vi "有限步数转动.vi"(8 "error in (no error)":errorcluster caption="错误输入（无错误）", 10 "samples per channel":i32=1000 caption="脉冲数", 11 "Hardware Resources in":T1 caption="硬件资源输入") -> (0 "error out":errorcluster caption="错误输出", 3 "Hardware Resources out":T1 caption="硬件资源输出")   [LabVIEW 2015, in "Action.lvlib"]
doc: "初始化硬件引用。"
uses:
  Action.lvlib
  <vilib>/DAQmx/create/channels.llb/DAQmx Create Channel (CO-Pulse Generation-Frequency).vi
  <vilib>/DAQmx/configure/timing.llb/DAQmx Timing (Implicit).vi
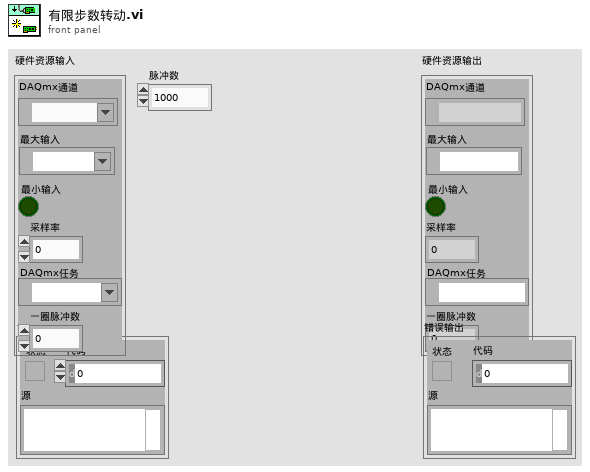
[diagram p1: front panel]
types:
  T1 = typedef "Action.lvlib/电机控制设置.ctl" = cluster{"counter":tag, "方向端口":tag, "当前方向":bool, "频率":dbl, "DAQmx Task":refnum<k21>, "一圈脉冲数":i32}
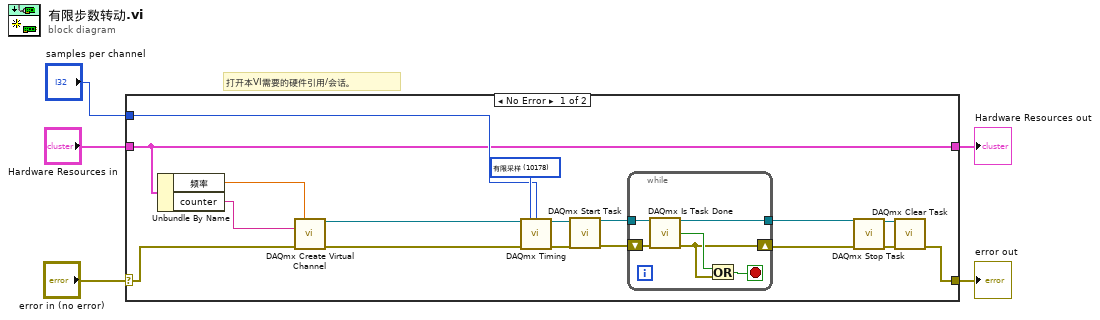
[diagram p0: block diagram]
diagram:
  # "打开本VI需要的硬件引用/会话。"
  n1 = case shown="No Error" "error in (no error)" {
    selector: "error in (no error)" -> [w6 w29]
    tunnel: [w20 w29] -> w4
    tunnel: "Hardware Resources in" -> [w15 w30]
    tunnel: [w15 w30] -> w2
    tunnel: "samples per channel" -> [w16 _]
    frame No Error {
      w17 = 10178 items=["有限采样"=10178, "连续采样"=10123, "硬件定时单点"=12522] ("sample mode")
      n2 = Unbundle By Name(w15) -> ("频率"=w18:dbl, "counter"=w19:tag)
      n3 = call-poly <vilib>:"DAQmx Create Virtual Channel.vi"("frequency"=w18, "counter"=w19, "error in"=w6) -> ("task out"=w8:refnum<k21>, "error out"=w7:errorcluster)  [unwired: 11 in]
      n4 = call-poly <vilib>:"DAQmx Timing.vi"("task/channels in"=w8, "sample mode"=w17, "samples per channel"=w16, "error in"=w7) -> ("task out"=w14:refnum<k21>, "error out"=w13:errorcluster)  [unwired: 10 in]
      n5 = call <vilib>:"DAQmx Start Task.vi"("task/channels in"=w14, "error in"=w13) -> ("task out"=w12:refnum<k21>, "error out"=w11:errorcluster)  [unwired: 12 in]
      n6 = while {
        tunnel: w12 -> [w28]
        shift-right: [w24] -> w9
        shift-left: w11 -> [w27]
        tunnel: [w23] -> w10
        stop <- w25 stop-if-true
        n7 = call <vilib>:"DAQmx Is Task Done.vi"("task/channels in"=w28, "error in"=w27) -> ("task out"=w23:refnum<k21>, "task done?"=w26:bool, "error out"=w24:errorcluster)  [unwired: 11 in]
        n8 = Or(x=w26, y=w24) -> (x .or. y?=w25:bool)
      }
      n9 = call <vilib>:"DAQmx Stop Task.vi"("task/channels in"=w10, "error in"=w9) -> ("task out"=w21:refnum<k21>, "error out"=w22:errorcluster)  [unwired: 12 in]
      n10 = call <vilib>:"DAQmx Clear Task.vi"("task in"=w21, "error in"=w22) -> ("error out"=w20:errorcluster)  [unwired: 13 in]
    }
    frame Error {
    }
  }
  "Hardware Resources out" <- w2
  "error out" <- w4
